vi "Random String__jki_lib_data_manipulation -- VI Tester.vi"(4 "length":i32) -> (1 "random data":string)   [LabVIEW 2011]
doc: "Outputs a <B>random data</B> string of the specified <B>length</B>."
panel:
  # "Copyright © 2006 James Kring, Inc. All rights reserved.\n\nThis library is provided \"AS IS\" , WITHOUT WARRANTIES OR \nCONDITIONS OF ANY KIND, either express or implied.\n\nJames Kring, Inc. -- http://www.jameskring.com"
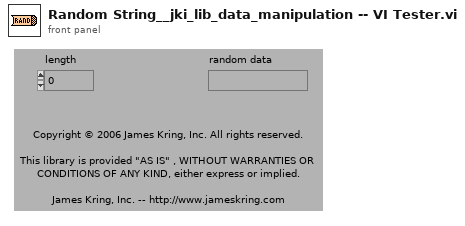
[diagram p1: front panel]
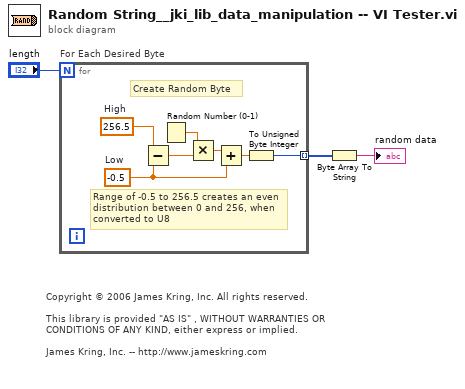
[diagram p0: block diagram]
diagram:
  # "Copyright © 2006 James Kring, Inc. All rights reserved.\n\nThis library is provided \"AS IS\" , WITHOUT WARRANTIES OR \nCONDITIONS OF ANY KIND, either express or implied.\n\nJames Kring, Inc. -- http://www.jameskring.com"
  n1 = for "For Each Desired Byte" {
    N: "length" -> [_]
    tunnel: [w10] -> w2 mode=indexing
    w5 = 256.5  # High
    w6 = -0.5  # Low
    # "Range of -0.5 to 256.5 creates an even distribution between 0 and 256, when converted to U8"
    # "Create Random Byte"
    n2 = Subtract(x=w5, y=w6) -> (x-y=w8:dbl)
    n3 = Random Number (0-1)() -> (number: 0 to 1=w7:dbl)
    n4 = Multiply(x=w7, y=w8) -> (x*y=w9:dbl)
    n5 = Add(x=w9, y=w6) -> (x+y=w4:dbl)
    n6 = To Unsigned Byte Integer(number=w4) -> (unsigned 8bit integer=w10:u8)
  }
  n7 = Byte Array To String(unsigned byte array=w2) -> (string=→"random data":string)
